vi "ExposeMapperDestroyValueNamepathDescriptionWithRefs.vi"(10 "Collect values":bool, 11 "NPDsc":T1[](array[typedef])) -> (3 "Values":variant[](array[variant]))   [LabVIEW 2017]
uses:
  ExposeMapperUpdateNamepathPartDescriptor.ctl
  ExposeMapperUpdateNamepathPartDescriptorEnum.ctl
  ExposeObjectMapContainerTypeEnum.ctl
  <userlib>/_OpenG.lib/array/array.llb/Conditional Auto-Indexing Tunnel (Variant)__ogtk.vi
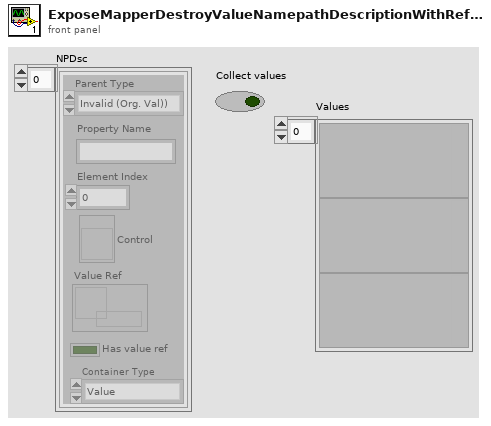
[diagram p1: front panel]
types:
  T1 = typedef "ExposeMapperUpdateNamepathPartDescriptor.ctl" = cluster{"Parent Type":T2, "Property Name":string, "Element Index":i32, "Control":refnum<vi>, "Value Ref":refnum<data-value>, "Has value ref":bool, "Container Type":T3}
  T2 = typedef "ExposeMapperUpdateNamepathPartDescriptorEnum.ctl" = enum16{"Invalid (Org. Val))", "Default Value", "Value", "Variant", "Cluster", "Array", "Refnum"}
  T3 = typedef "ExposeObjectMapContainerTypeEnum.ctl" = enum16{"Value", "Array", "Waveform", "NetContainer"}
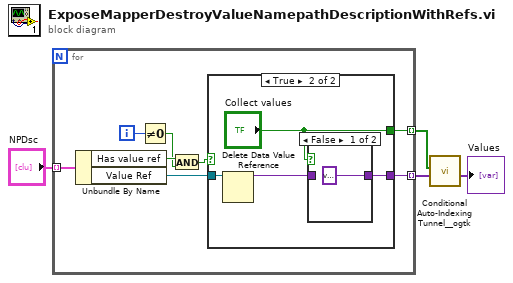
[diagram p0: block diagram]
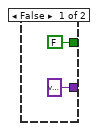
[diagram p2: hidden frame]
diagram:
  n1 = for {
    tunnel: "NPDsc" -> [w11] mode=indexing
    tunnel: [w6] -> w3 mode=indexing
    tunnel: [w5] -> w2 mode=indexing
    i -> [w12]
    n2 = Unbundle By Name(w11) -> ("Has value ref"=w9:bool, "Value Ref"=w7:refnum<data-value>)
    n3 = Not Equal To 0?(x=w12) -> (x != 0?=w8:bool)
    n4 = And(x=w9, y=w8) -> (x .and. y?=w10:bool)
    n5 = case shown="True" w10 {
      tunnel: w7 -> [_ w18]
      tunnel: [FALSE ("Collect values") "Collect values"] -> w6
      tunnel: [variant ("Array") w16] -> w5
      frame False {
      }
      frame True {
        n6 = Delete Data Value Reference(data value reference=w18) -> (data value=w17:variant)  [unwired: 1 in, 1 out]
        n7 = case shown="False" "Collect values" {
          tunnel: w17 -> [_ w20]
          tunnel: [variant ("Array") w20] -> w16
          frame False {
          }
          frame True {
          }
        }
      }
    }
  }
  n8 = call-poly <userlib>:"Conditional Auto-Indexing Tunnel__ogtk.vi"("Array in"=w2, "Elements to keep"=w3) -> ("Filtered Array out"=→"Values":variant[])  [unwired: 5 in]
